vi "LvMPDC_CMD_option_random.vi"(6 "timeout_ms":i32=3000, 8 "error in (no error)":errorcluster, 9 "ReadBytes":i32=1024, 10 "sw":bool, 11 "Connect ID":refnum<k5>) -> (0 "error out":errorcluster, 3 "Connect ID out":refnum<k5>)   [LabVIEW 2012]
panel:
  # "LvMPDC:: CMD random (playback option)"
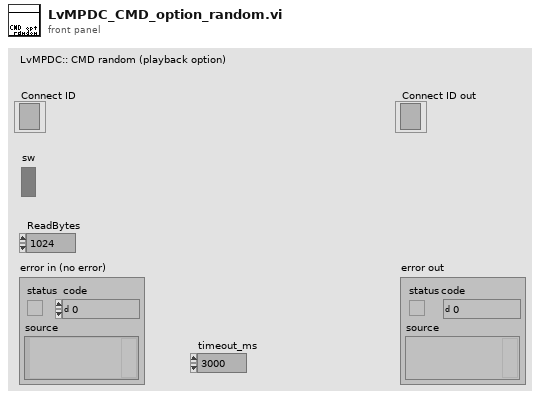
[diagram p1: front panel]
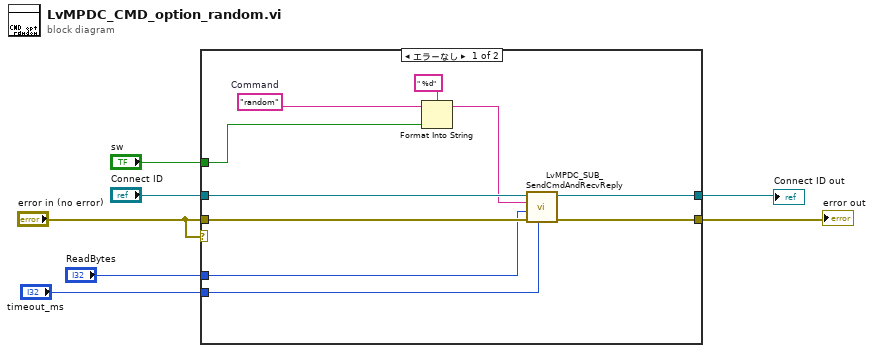
[diagram p0: block diagram]
diagram:
  n1 = case shown="エラーなし" "error in (no error)" {
    tunnel: "Connect ID" -> [w15 w19]
    tunnel: "error in (no error)" -> [w17 w18]
    tunnel: [w14 w19] -> w6
    tunnel: [w16 w18] -> w5
    tunnel: "timeout_ms" -> [w12 _]
    tunnel: "ReadBytes" -> [w13 _]
    tunnel: "sw" -> [w8 _]
    frame No Error {
      w11 = "random"  # Command
      n2 = Format Into String(format string=" %d" ("形式文字列"), initial string=w11, w8) -> (resulting string=w9:string)  [unwired: 1 in, 1 out]
      n3 = call "LvMPDC_SUB_SendCmdAndRecvReply.vi"("timeout_ms"=w12, "error in (no error)"=w17, "ReadBytes"=w13, "Command"=w9, "Connect ID"=w15) -> ("error out"=w16:errorcluster, "Connect ID out"=w14:refnum<k5>)  [unwired: 4 in, 1 out]
    }
    frame Error {
    }
  }
  "Connect ID out" <- w6
  "error out" <- w5
